vi "Get Model Roll Pitch Yaw.vi"(2 "Mode":T1, 3 "Traverse Name":string) -> (0 "Traverse origin x offset":sgl, 1 "Model:    Roll        Pitch         Yaw  (deg)":sgl[](array[numeric]) caption="ModelRollPitchYaw (deg)" format="%#.2f")   [LabVIEW 2017]
uses:
  Controls/User_Specific_mode.ctl
  ADAM Client/Sub VIs/ADAM Controls/Quick_local_ADAM_Table.ctl
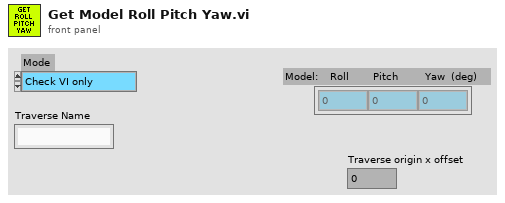
[diagram p1: front panel]
types:
  T1 = typedef "User_Specific_mode.ctl" = enum16{"Check VI only", "Run VI"}
  T2 = typedef "Quick_local_ADAM_Table.ctl" = enum16{"Read Global", "Load Global From ADAM Table", "Write Global"}
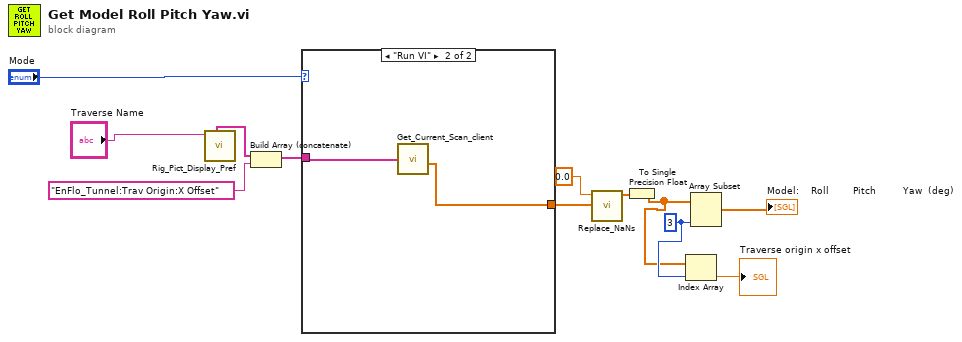
[diagram p0: block diagram]
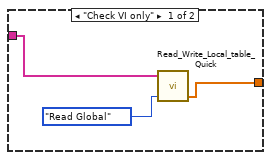
[diagram p2: hidden frame]
diagram:
  w11 = 3 ("length")
  n1 = call "Rig_Pict_Display_Pref.vi"("Traverse Name"="Traverse Name") -> ("Roll Pitch Yaw ADAM Channels"=w7:string[])  [unwired: 3 in, 4 out]
  n2 = Build Array (concatenate)(w7, "EnFlo_Tunnel:Trav Origin:X Offset") -> (w9:string[])
  n3 = case shown="\"Run VI\"" "Mode" {
    tunnel: [w14 w16] -> w4
    tunnel: w9 -> [w15 w17]
    frame "Check VI only" {
      n4 = call "Read_Write_Local_table_Quick.vi"("Mode"=Quick_local_ADAM_Table."Read Global", "Ch names In"=w15) -> ("Numeric Values Out"=w14:dbl[])  [unwired: 1 in, 2 out]
    }
    frame "Run VI" {
      n5 = call "Get_Current_Scan_client.vi"("ADAM Ch Names"=w17) -> ("Numerical Values"=w16:dbl[])  [unwired: 3 out]
    }
  }
  n6 = call "Replace_NaNs.vi"("Array"=w4, "Replacement"=0.0) -> ("Array Out"=w6:dbl[])  [unwired: 9 in]
  n7 = To Single Precision Float(number=w6) -> (single precision float=w10:sgl[])
  n8 = Index Array(array=w10, index=w11) -> (element=→"Traverse origin x offset":sgl)
  n9 = Array Subset(array=w10, length=w11) -> (→"Model:    Roll        Pitch         Yaw  (deg)":sgl[])  [unwired: 1 in]
